vi "RichToFlathelloworld_HelloRequest.vi"(5 "OutputClusterType":T1, 11 "InputCluster":T2) -> (3 "OutputCluster":T1)   [LabVIEW 2019, in "helloworld_client.lvlib"]
uses:
  helloworld_client.lvlib
  helloworld_HelloRequest.ctl
  helloworld_HelloRequest_Flat.ctl
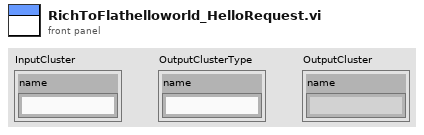
[diagram p1: front panel]
types:
  T1 = typedef "helloworld_client.lvlib/helloworld_HelloRequest_Flat.ctl" = cluster{"name":string}
  T2 = typedef "helloworld_client.lvlib/helloworld_HelloRequest.ctl" = cluster{"name":string}
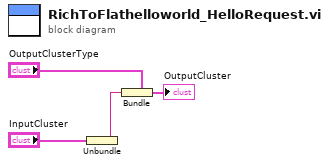
[diagram p0: block diagram]
diagram:
  n1 = Unbundle "Unbundle"("InputCluster") -> ("name"=w1:string)
  n2 = Bundle "Bundle"(cluster="OutputClusterType", "name"=w1) -> (→"OutputCluster":T1)
